vi "Configure Modulation (Burst).vi"(0 "VISA resource name":refnum<visa-resource-name>, 1 "Burst Phase (0 deg)":i32 min=-360 max=360, 2 "Burst Count (1)":i32=1, 3 "Burst Period (1 s)":dbl=1.0 min=0.002 max=1000000.0 format="%.6f", 5 "Enable Burst Modulation (T: Enable)":bool=TRUE, 7 "Burst Modulation Mode (0: Triggered)":u16(ring) items=["Triggered", "Gated"], 11 "error in (no error)":errorcluster) -> (4 "VISA resource name out":refnum<visa-resource-name>, 15 "error out":errorcluster)   [LabVIEW 2026, in "Agilent 33XXX Series.lvlib"]
doc: "Allows and configures burst modulation. Configures the function generator to output a waveform with specified number of cycles, called burst. The carrier waveform shape and parameters are set by Configure Standard Waveform.\n\nNote:\n(1) Before using this mode, all other modes must be turned off.\n(2) This VI is not valid in 33210."
uses:
  Agilent 33XXX Series.lvlib
panel:
  # "Triggered BM Settings"
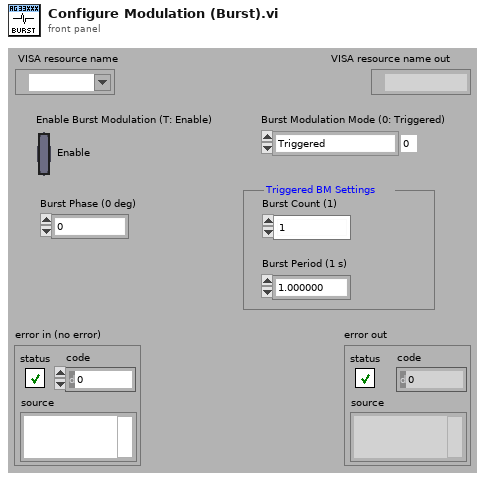
[diagram p1: front panel]
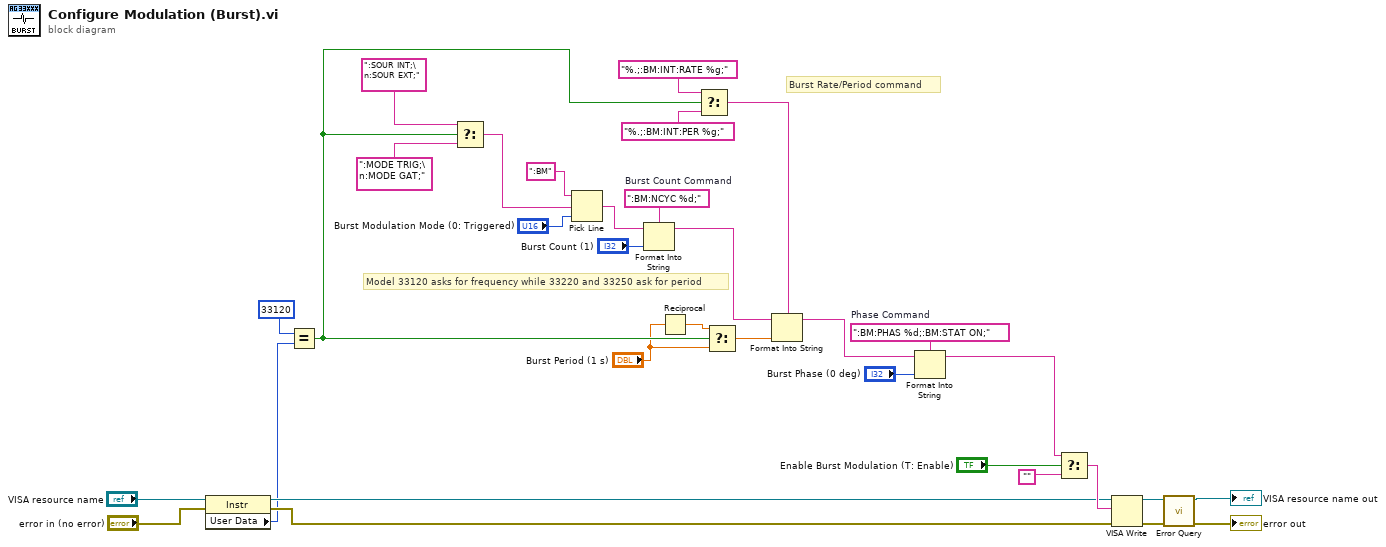
[diagram p0: block diagram]
diagram:
  w30 = ":BM:PHAS %d;:BM:STAT ON;"  # Phase Command
  w31 = ":BM:NCYC %d;"  # Burst Count Command
  # "Model 33120 asks for frequency while 33220 and 33250 ask for period"
  # "Burst Rate/Period command"
  n1 = property class="Instr"(reference="VISA resource name", error in="error in (no error)") -> (reference out=w24:refnum<visa-resource-name>, error out=w23:errorcluster, "User Data"=w22:u32)
  n2 = Equal?(x=u32 33120, y=w22) -> (x = y?=w13:bool)
  n3 = Select(t=":SOUR INT;\n:SOUR EXT;" ("Source Command"), s=w13, f=":MODE TRIG;\n:MODE GAT;") -> (s? t:f=w18:string)
  n4 = Pick Line(string ("")=":BM", multi-line string=w18, line index="Burst Modulation Mode (0: Triggered)") -> (output string=w17:string)
  n5 = Format Into String(format string=w31, initial string=w17, "Burst Count (1)") -> (resulting string=w9:string)  [unwired: 1 in, 1 out]
  n6 = Reciprocal(x="Burst Period (1 s)") -> (1/x=w12:dbl)
  n7 = Select(t="%.;:BM:INT:RATE %g;" ("Rate Command"), s=w13, f="%.;:BM:INT:PER %g;") -> (s? t:f=w14:string)
  n8 = Select(t=w12, s=w13, f="Burst Period (1 s)") -> (s? t:f=w10:dbl)
  n9 = Format Into String(format string=w14, initial string=w9, w10) -> (resulting string=w8:string)  [unwired: 1 in, 1 out]
  n10 = Format Into String(format string=w30, initial string=w8, "Burst Phase (0 deg)") -> (resulting string=w7:string)  [unwired: 1 in, 1 out]
  n11 = Select(t=w7, s="Enable Burst Modulation (T: Enable)", f="") -> (s? t:f=w27:string)
  n12 = VISA Write(VISA resource name=w24, write buffer=w27, error in (no error)=w23) -> (VISA resource name out=w33:refnum<visa-resource-name>, error out=w32:errorcluster)  [unwired: 1 out]
  n13 = call "Error Query.vi"("error in (no error)"=w32, "VISA resource name"=w33) -> ("error out"=→"error out":errorcluster, "VISA resource name out"=→"VISA resource name out":refnum<visa-resource-name>)  [unwired: 6 in, 2 out]
